vi "Move All Selected.vi"(8 "error in (no error)":errorcluster, 10 "Delta":T1, 11 "Editor Handler in":refnum<class "Image Editor Handler.lvclass">) -> (0 "error out":errorcluster, 3 "Editor Handler out":refnum<class "Image Editor Handler.lvclass">)   [LabVIEW 2015, in "LV Image Editor Framework.lvlib" / "Image Editor Handler.lvclass"]
uses:
  Image Editor Handler.lvclass
  <vilib>/Utility/miscctls.llb/LVPoint32TypeDef.ctl
  Image Editor Handler.lvclass/Image Editor Handler.ctl
  Forms/Shape/Shape.lvclass
  Image/Image.lvclass
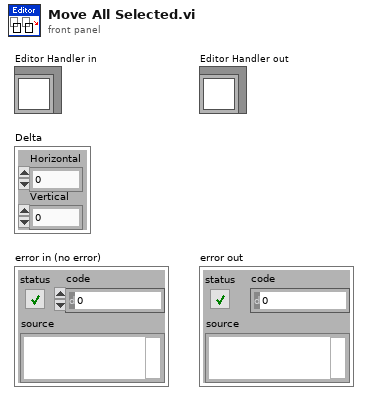
[diagram p1: front panel]
types:
  T1 = typedef "LVPoint32TypeDef.ctl" = cluster{"Horizontal":i32, "Vertical":i32}
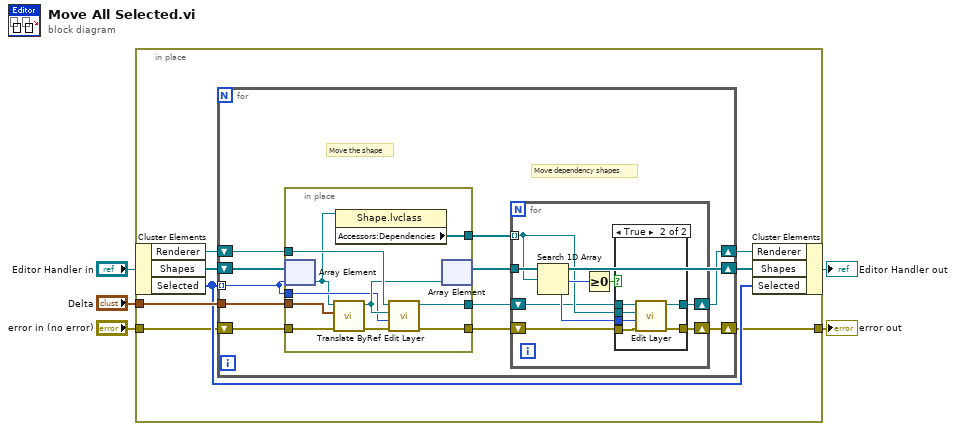
[diagram p0: block diagram]
diagram:
  n1 = in-place {
    in-place-border: "Delta" -> [w12]
    in-place-border: "error in (no error)" -> [w8]
    in-place-border: [w7] -> w5
    n2 = in-place-cluster #1("Editor Handler in") -> ("Renderer"=w9:refnum<class "Image.lvclass">, "Shapes"=w13:refnum<data-value>[], "Selected"=w10:i16[])
    n3 = for {
      tunnel: w10 -> [w22] mode=indexing
      tunnel: w12 -> [w24]
      shift-right: [w19] -> w11
      shift-left: w13 -> [w20]
      shift-right: [w16] -> w6
      shift-left: w9 -> [w23]
      shift-right: [w15] -> w7
      shift-left: w8 -> [w21]
      # "Move the shape"
      # "Move dependency shapes"
      n4 = in-place {
        in-place-border: w24 -> [w34]
        in-place-border: w23 -> [w33]
        in-place-border: [w32] -> w17
        in-place-border: w22 -> [w30]
        in-place-border: w21 -> [w28]
        in-place-border: [w27] -> w14
        in-place-border: [w26] -> w18
        n5 = in-place-array #2(w20, w22) -> (w25:refnum<data-value>)
        n6 = call "Translate ByRef.vi"("error in (no error)"=w28, "Translation"=w34, "ShapeRef"=w25) -> ("error out"=w29:errorcluster, "ShapeRef Out"=w31:refnum<data-value>)  [unwired: 7 in]
        n7 = property class="Shape.lvclass"(reference=w25) -> ("Accessors:Dependencies"=w26:refnum<data-value>[])  [unwired: 1 in, 2 out]
        n8 = call "Edit Layer.vi"("error in (no error)"=w29, "Layer Index"=w30, "ShapeRef"=w31, "Image in"=w33) -> ("error out"=w27:errorcluster, "Image out"=w32:refnum<class "Image.lvclass">)  [unwired: 6 in]
        n9 = in-place-array #2(w31) -> (w19:refnum<data-value>[])  [unwired: 1 out]
      }
      n10 = for {
        tunnel: w19 -> [w42]
        tunnel: w18 -> [w39] mode=indexing
        shift-right: [w37] -> w16
        shift-left: w17 -> [w38]
        shift-right: [w36] -> w15
        shift-left: w14 -> [w35]
        n11 = Search 1D Array(1D array=w42, element=w39) -> (index of element=w40:i32)  [unwired: 1 in]
        n12 = Greater Or Equal To 0?(x=w40) -> (x >= 0?=w41:bool)
        n13 = case shown="True" w41 {
          tunnel: w40 -> [_ w50]
          tunnel: w39 -> [_ w49]
          tunnel: w38 -> [w44 w48]
          tunnel: [w44 w47] -> w37
          tunnel: [w43 w46] -> w36
          tunnel: w35 -> [w43 w45]
          frame False {
          }
          frame True {
            n14 = call "Edit Layer.vi"("error in (no error)"=w45, "Layer Index"=w50, "ShapeRef"=w49, "Image in"=w48) -> ("error out"=w46:errorcluster, "Image out"=w47:refnum<class "Image.lvclass">)  [unwired: 6 in]
          }
        }
      }
    }
    n15 = in-place-cluster #1("Renderer"=w6, "Shapes"=w11, "Selected"=w10) -> (→"Editor Handler out":refnum<class "Image Editor Handler.lvclass">)
  }
  "error out" <- w5
